vi "nirviVBlockImpl.vi"   [LabVIEW 2017]
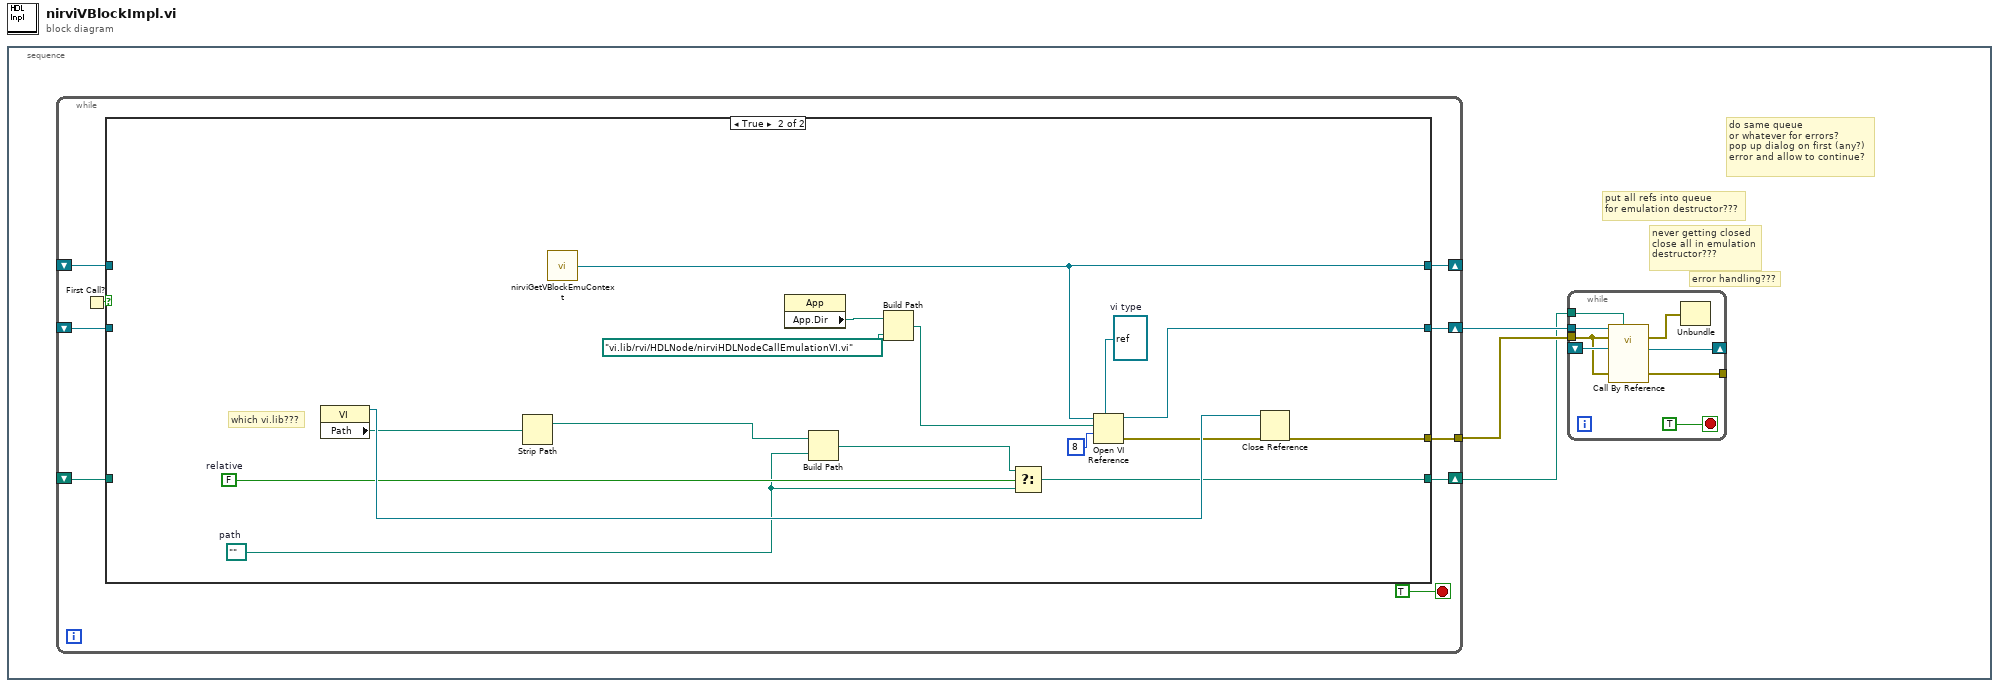
[diagram p0: block diagram]
diagram:
  n1 = stacked-sequence {
    frame #0 {
      # "do same queue\nor whatever for errors?\npop up dialog on first (any?)\nerror and allow to continue?"
      # "put all refs into queue\nfor emulation destructor???"
      # "never getting closed\nclose all in emulation\ndestructor???"
      # "error handling???"
      n2 = while {
        shift-right: [w17] -> _
        shift-left: _ -> [w18]
        shift-right: [w15] -> w3
        shift-left: _ -> [w14]
        tunnel: [w16] -> w2
        shift-right: [w13] -> w1
        shift-left: _ -> [w12]
        stop <- TRUE stop-if-true
        n3 = First Call?() -> (First Call?: T/F=w19:bool)
        n4 = case shown="True" w19 {
          tunnel: w18 -> [w23 _]
          tunnel: [w23 w24] -> w17
          tunnel: [_ w38] -> w16
          tunnel: [w22 w32] -> w15
          tunnel: w14 -> [w22 _]
          tunnel: [w21 w26] -> w13
          tunnel: w12 -> [w21 _]
          frame False {
          }
          frame True {
            w39 = refnum<vi> refnum  # vi type
            w33 = path ""  # path
            w35 = FALSE  # relative
            # "which vi.lib???"
            n5 = property class="VI"() -> (reference out=w37:refnum<vi>, "Path"=w34:path)  [unwired: 2 in, 1 out]
            n6 = Strip Path(path=w34) -> (stripped path=w30:path)  [unwired: 1 out]
            n7 = call <vilib>:"nirviGetVBlockEmuContext.vi"() -> ("context"=w24:refnum<vi>)
            n8 = property class="App"() -> ("App.Dir"=w29:path)  [unwired: 2 in, 2 out]
            n9 = Build Path(base path=w30, name or relative path=w33) -> (appended path=w36:path)
            n10 = Build Path(base path=w29, name or relative path=path "vi.lib/rvi/HDLNode/nirviHDLNodeCallEmulationVI.vi" ("Application:Directory Path")) -> (appended path=w27:path)
            n11 = Select(t=w36, s=w35, f=w33) -> (s? t:f=w26:path)
            n12 = Open VI Reference(type specifier VI Refnum (for type only)=w39, application reference (local)=w24, vi path=w27, options=8) -> (vi reference=w32:refnum<vi>, error out=w31:errorcluster)  [unwired: 1 in, 1 out]
            n13 = Close Reference(reference=w37, error in (no error)=w31) -> (error out=w38:errorcluster)
          }
        }
      }
      n14 = while {
        tunnel: w3 -> [w11]
        tunnel: w2 -> [w5]
        tunnel: w1 -> [w9]
        shift-right: [w7] -> _
        shift-left: _ -> [w8]
        tunnel: [w4] -> _
        stop <- TRUE stop-if-true
        n15 = call-by-ref "?"(reference=w11, error in=w5, "vi reference in"=w8, "Emulation VI Location"=w9, "error in (no error)"=w5) -> (error out=w10:errorcluster, "vi reference"=w7:refnum<vi>, 15:"error out"=w4:errorcluster)  [unwired: 10 in, 2 out]
        n16 = Unbundle(w10) -> ()  [unwired: 3 out]
      }
    }
  }
